vi "PCA.vi"(8 "error in":errorcluster) -> (0 "error out":errorcluster, 3 "out":refnum<class "PCA.lvclass">)   [LabVIEW 2020]
doc: "Principal component analysis (PCA).\n\n Linear dimensionality reduction using Singular Value Decomposition of the\n data to project it to a lower dimensional space. The input data is centered\n but not scaled for each feature before applying the SVD.\n\n It uses the LAPACK implementation of the full SVD or a randomized truncated\n SVD by the method of Halko et al. 2009, depending on the shape of the input\n data and the number of components to extract.\n\n It can also use the scipy.sparse.linalg ARPACK implementation of the\n truncated SVD.\n\n Notice that this class does not support sparse input. See\n :class:`TruncatedSVD` for an alternative with sparse data.\n\n Read more in the :ref:`User Guide <PCA>`.\n\n Parameters\n ----------\n n_components : int, float or 'mle', default=None\n Number of components to keep.\n if n_components is not set all components are kept::\n\n n_components == min(n_samples, n_features)\n\n If ``n_components == 'mle'`` and ``svd_solver == 'full'``, Minka's\n MLE is used to guess the dimension. Use of ``n_components == 'mle'``\n will interpret ``svd_solver == 'auto'`` as ``svd_solver == 'full'``.\n\n If ``0 < n_components < 1`` and ``svd_solver == 'full'``, select the\n number of components such that the amount of variance that needs to be\n explained is greater than the percentage specified by n_components.\n\n If ``svd_solver == 'arpack'``, the number of components must be\n strictly less than the minimum of n_features and n_samples.\n\n Hence, the None case results in::\n\n n_components == min(n_samples, n_features) - 1\n\n copy : bool, default=True\n If False, data passed to fit are overwritten and running\n fit(X).transform(X) will not yield the expected results,\n use fit_transform(X) instead.\n\n whiten : bool, default=False\n When True (False by default) the `components_` vectors are multiplied\n by the square root of n_samples and then divided by the singular values\n to ensure uncorrelated outputs with unit component-wise variances.\n\n Whitening will remove some information from the transformed signal\n (the relative variance scales of the components) but can sometime\n improve the predictive accuracy of the downstream estimators by\n making their data respect some hard-wired assumptions.\n\n svd_solver : {'auto', 'full', 'arpack', 'randomized'}, default='auto'\n If auto :\n The solver is selected by a default policy based on `X.shape` and\n `n_components`: if the input data is larger than 500x500 and the\n number of components to extract is lower than 80% of the smallest\n dimension of the data, then the more efficient 'randomized'\n method is enabled. Otherwise the exact full SVD is computed and\n optionally truncated afterwards.\n If full :\n run exact full SVD calling the standard LAPACK solver via\n `scipy.linalg.svd` and select the components by postprocessing\n If arpack :\n run SVD truncated to n_components calling ARPACK solver via\n `scipy.sparse.linalg.svds`. It requires strictly\n 0 < n_components < min(X.shape)\n If randomized :\n run randomized SVD by the method of Halko et al.\n\n .. versionadded:: 0.18.0\n\n tol : float, default=0.0\n Tolerance for singular values computed by svd_solver == 'arpack'.\n Must be of range [0.0, infinity).\n\n .. versionadded:: 0.18.0\n\n iterated_power : int or 'auto', default='auto'\n Number of iterations for the power method computed by\n svd_solver == 'randomized'.\n Must be of range [0, infinity).\n\n .. versionadded:: 0.18.0\n\n random_state : int, RandomState instance or None, default=None\n Used when the 'arpack' or 'randomized' solvers are used. Pass an int\n for reproducible results across multiple function calls.\n See :term:`Glossary <random_state>`.\n\n .. versionadded:: 0.18.0\n\n Attributes\n ----------\n components_ : ndarray of shape (n_components, n_features)\n Principal axes in feature space, representing the directions of\n maximum variance in the data. The components are sorted by\n ``explained_variance_``.\n\n explained_variance_ : ndarray of shape (n_components,)\n The amount of variance explained by each of the selected components.\n The variance estimation uses `n_samples - 1` degrees of freedom.\n\n Equal to n_components largest eigenvalues\n of the covariance matrix of X.\n\n .. versionadded:: 0.18\n\n explained_variance_ratio_ : ndarray of shape (n_components,)\n Percentage of variance explained by each of the selected components.\n\n If ``n_components`` is not set then all components are stored and the\n sum of the ratios is equal to 1.0.\n\n singular_values_ : ndarray of shape (n_components,)\n The singular values corresponding to each of the selected components.\n The singular values are equal to the 2-norms of the ``n_components``\n variables in the lower-dimensional space.\n\n .. versionadded:: 0.19\n\n mean_ : ndarray of shape (n_features,)\n Per-feature empirical mean, estimated from the training set.\n\n Equal to `X.mean(axis=0)`.\n\n n_components_ : int\n The estimated number of components. When n_components is set\n to 'mle' or a number between 0 and 1 (with svd_solver == 'full') this\n number is estimated from input data. Otherwise it equals the parameter\n n_components, or the lesser value of n_features and n_samples\n if n_components is None.\n\n n_features_ : int\n Number of features in the training data.\n\n n_samples_ : int\n Number of samples in the training data.\n\n noise_variance_ : float\n The estimated noise covariance following the Probabilistic PCA model\n from Tipping and Bishop 1999. See \"Pattern Recognition and\n Machine Learning\" by C. Bishop, 12.2.1 p. 574 or\n http://www.miketipping.com/papers/met-mppca.pdf. It is required to\n compute the estimated data covariance and score samples.\n\n Equal to the average of (min(n_features, n_samples) - n_components)\n smallest eigenvalues of the covariance matrix of X.\n\n See Also\n --------\n KernelPCA : Kernel Principal Component Analysis.\n SparsePCA : Sparse Principal Component Analysis.\n TruncatedSVD : Dimensionality reduction using truncated SVD.\n IncrementalPCA : Incremental Principal Component Analysis.\n\n References\n ----------\n For n_components == 'mle', this class uses the method from:\n `Minka, T. P.. \"Automatic choice of dimensionality for PCA\".\n In NIPS, pp. 598-604 <https://tminka.github.io/papers/pca/minka-pca.pdf>`_\n\n Implements the probabilistic PCA model from:\n `Tipping, M. E., and Bishop, C. M. (1999). \"Probabilistic principal\n component analysis\". Journal of the Royal Statistical Society:\n Series B (Statistical Methodology), 61(3), 611-622.\n <http://www.miketipping.com/papers/met-mppca.pdf>`_\n via the score and score_samples methods.\n\n For svd_solver == 'arpack', refer to `scipy.sparse.linalg.svds`.\n\n For svd_solver == 'randomized', see:\n `Halko, N., Martinsson, P. G., and Tropp, J. A. (2011).\n \"Finding structure with randomness: Probabilistic algorithms for\n constructing approximate matrix decompositions\".\n SIAM review, 53(2), 217-288.\n <https://doi.org/10.1137/090771806>`_\n and also\n `Martinsson, P. G., Rokhlin, V., and Tygert, M. (2011).\n \"A randomized algorithm for the decomposition of matrices\".\n Applied and Computational Harmonic Analysis, 30(1), 47-68\n <https://doi.org/10.1016/j.acha.2010.02.003>`_.\n\n \nAvailable methods:\nFit\nFit Transform\nTransform\nGet Attributes\nGet Params\nSet Params"
uses:
  PCA.lvclass
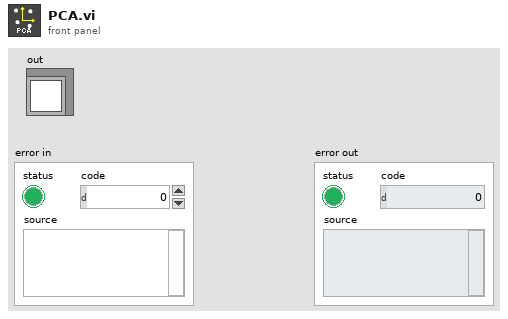
[diagram p1: front panel]
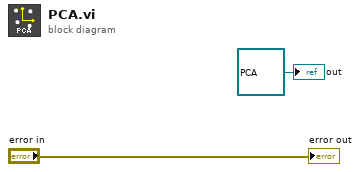
[diagram p0: block diagram]
diagram:
  "out" <- refnum<class "PCA.lvclass"> refnum ("model")
  "error out" <- "error in"
